vi "Save Local Personality File.vi"(8 "error in (no error)":errorcluster, 10 "New Content":string, 11 "File Path":path) -> (0 "error out":errorcluster, 3 "Path out":path)   [LabVIEW 2018, in "Personalities Tool.lvlib"]
doc: "This VI takes a file path and replaces the contents for the ones yoiu send in the input string."
uses:
  Personalities Tool.lvlib
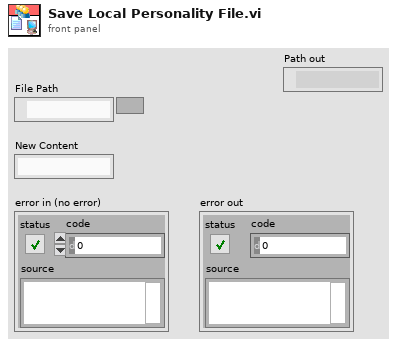
[diagram p1: front panel]
types:
  T1 = enum16{"open", "replace", "create", "open or create", "replace or create", "replace or create with confirmation"}
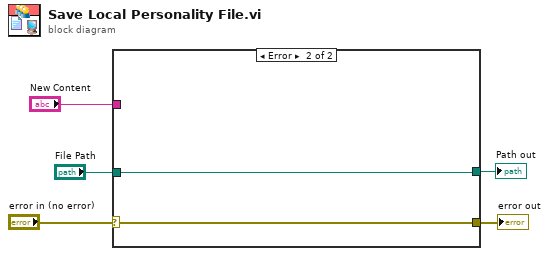
[diagram p0: block diagram]
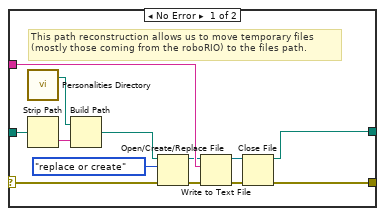
[diagram p2: hidden frame]
diagram:
  n1 = case shown="Error" "error in (no error)" {
    selector: "error in (no error)" -> [w15 w20]
    tunnel: [w18 w20] -> w5
    tunnel: "New Content" -> [w16 _]
    tunnel: "File Path" -> [w10 w19]
    tunnel: [w6 w19] -> w1
    frame No Error {
      # "This path reconstruction allows us to move temporary files\n(mostly those coming from the roboRIO) to the files path."
      n2 = call "Personalities Directory.vi"() -> ("appended path"=w9:path)  [unwired: 3 in]
      n3 = Strip Path(path=w10) -> (name=w8:string)  [unwired: 1 out]
      n4 = Build Path(base path=w9, name or relative path=w8) -> (appended path=w7:path)
      n5 = Open/Create/Replace File(file path (use dialog)=w7, error in=w15, operation (0:open)=T1."replace or create") -> (refnum out=w11:refnum<file>, error out=w12:errorcluster)  [unwired: 3 in, 1 out]
      n6 = Write to Text File(file (use dialog)=w11, text=w16, error in=w12) -> (refnum out=w13:refnum<file>, error out=w14:errorcluster)  [unwired: 1 in, 1 out]
      n7 = Close File(refnum=w13, error in=w14) -> (path=w6:path, error out=w18:errorcluster)
    }
    frame Error {
    }
  }
  "error out" <- w5
  "Path out" <- w1
